vi "XMOLEdll.vi"(8 "error in (no error)":errorcluster, 11 "xkg":dbl[](array[numeric])) -> (0 "error out":errorcluster, 2 "wmix out":dbl, 3 "xmol out":dbl[](array[numeric]))   [LabVIEW 2016]
doc: "subroutine XMOLE (xkg,xmol,wmix)\n\nConverts composition on a mass fraction basis to mole fraction\n\nINPUTS:\n xkg--composition array [array of mass frac]\n\nOUTPUTS:\n xmol--composition array [array of mol frac]\n wmix--molar mass of the mixture [g/mol], a.k.a. \"molecular weight\""
uses:
  REFPROP.DLL
panel:
  # "REFPROP-XMOLEdll.vi"
  # "void  XMOLEdll(double *xkg, double *xmol, double *wmix)"
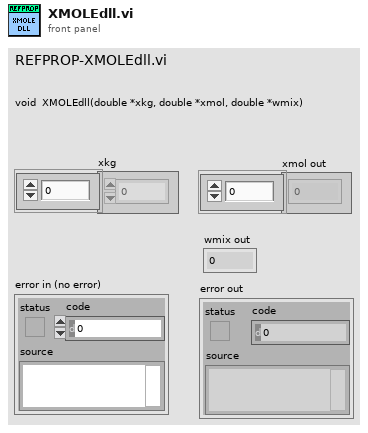
[diagram p1: front panel]
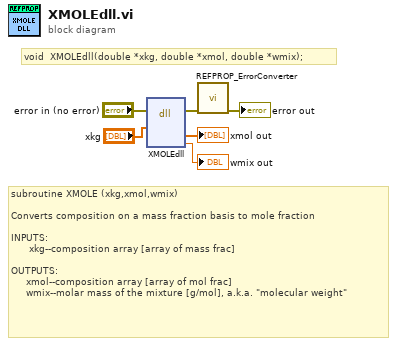
[diagram p0: block diagram]
diagram:
  # "void  XMOLEdll(double *xkg, double *xmol, double *wmix);"
  # "subroutine XMOLE (xkg,xmol,wmix)\n\nConverts composition on a mass fraction basis to mole fraction\n\nINPUTS:\n      xkg--composition array [array of mass frac]\n\nOUTPUTS:\n     xmol--composition array [array of mol frac]\n     wmix--molar mass of the mixture [g/mol], a.k.a. \"molecular weight\""
  n1 = dll-call lib="S:/009 - Testing/02 - Performance Testing/REFPROP/REFPROP.*" fn="XMOLEdll"(error in="error in (no error)", "xkg"="xkg") -> (error out=w3:errorcluster, "xmol"=→"xmol out":dbl[], "wmix"=→"wmix out":dbl)  [unwired: 6 in, 1 out]
  n2 = call "REFPROP_ErrorConverter.vi"("error in (no error)"=w3) -> ("error out"=→"error out":errorcluster)  [unwired: 10 in]
